vi "indicator.vi"(0 "Dial":i8(knob) scale=0.0..9.0, 1 "Boolean 9":bool) -> ()   [LabVIEW 2022 SP3]
panel:
  in  "stop":bool
  out "Boolean 8":bool
  out "Boolean 7":bool
  out "Boolean 6":bool
  out "Boolean 5":bool
  out "Boolean 4":bool
  out "Boolean 3":bool
  out "Boolean 2":bool
  out "Boolean":bool
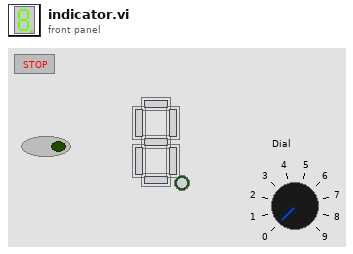
[diagram p1: front panel]
types:
  T1 = cluster{bool, bool, bool, bool, bool, bool, bool}
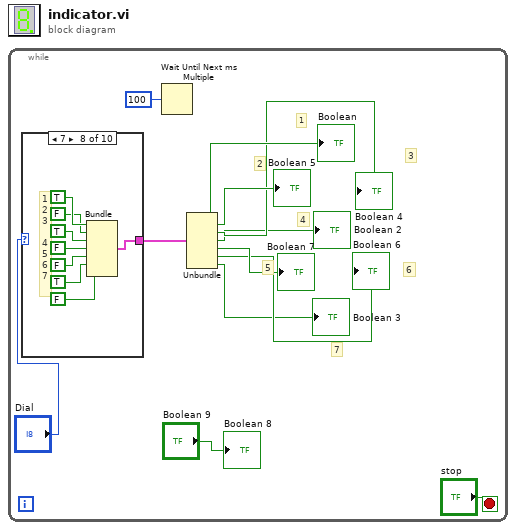
[diagram p0: block diagram]
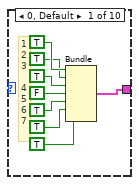
[diagram p2: hidden frame]
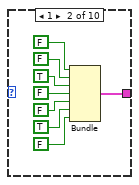
[diagram p3: hidden frame]
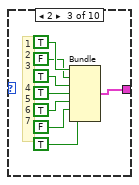
[diagram p4: hidden frame]
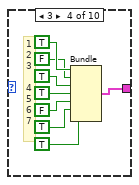
[diagram p5: hidden frame]
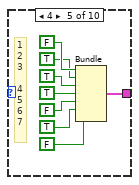
[diagram p6: hidden frame]
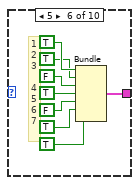
[diagram p7: hidden frame]
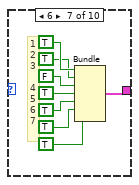
[diagram p8: hidden frame]
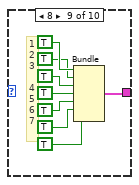
[diagram p9: hidden frame]
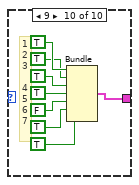
[diagram p10: hidden frame]
diagram:
  n1 = while {
    stop <- "stop" stop-if-true
    # "7"
    # "6"
    # "5"
    # "4"
    # "3"
    # "2"
    # "1"
    n2 = case shown="7" "Dial" {
      tunnel: [w13 w21 w29 w37 w45 w53 w61 w69 w77 w85] -> w12
      frame 0, Default {
        # "1\n2\n3\n\n4\n5\n6\n7"
        n3 = Bundle(TRUE, TRUE, TRUE, FALSE, TRUE, TRUE, TRUE) -> (w13:T1)  [unwired: 1 in]
      }
      frame 1 {
        n4 = Bundle(FALSE, FALSE, TRUE, FALSE, FALSE, TRUE, FALSE) -> (w21:T1)  [unwired: 1 in]
      }
      frame 2 {
        # "1\n2\n3\n\n4\n5\n6\n7"
        n5 = Bundle(TRUE, FALSE, TRUE, TRUE, TRUE, FALSE, TRUE) -> (w29:T1)  [unwired: 1 in]
      }
      frame 3 {
        # "1\n2\n3\n\n4\n5\n6\n7"
        n6 = Bundle(TRUE, FALSE, TRUE, TRUE, FALSE, TRUE, TRUE) -> (w37:T1)  [unwired: 1 in]
      }
      frame 4 {
        # "1\n2\n3\n\n4\n5\n6\n7"
        n7 = Bundle(FALSE, TRUE, TRUE, TRUE, FALSE, TRUE, FALSE) -> (w45:T1)  [unwired: 1 in]
      }
      frame 5 {
        # "1\n2\n3\n\n4\n5\n6\n7"
        n8 = Bundle(TRUE, TRUE, FALSE, TRUE, FALSE, TRUE, TRUE) -> (w53:T1)  [unwired: 1 in]
      }
      frame 6 {
        # "1\n2\n3\n\n4\n5\n6\n7"
        n9 = Bundle(TRUE, TRUE, FALSE, TRUE, TRUE, TRUE, TRUE) -> (w61:T1)  [unwired: 1 in]
      }
      frame 7 {
        # "1\n2\n3\n\n4\n5\n6\n7"
        n10 = Bundle(TRUE, FALSE, TRUE, FALSE, FALSE, TRUE, FALSE) -> (w69:T1)  [unwired: 1 in]
      }
      frame 8 {
        # "1\n2\n3\n\n4\n5\n6\n7"
        n11 = Bundle(TRUE, TRUE, TRUE, TRUE, TRUE, TRUE, TRUE) -> (w77:T1)  [unwired: 1 in]
      }
      frame 9 {
        # "1\n2\n3\n\n4\n5\n6\n7"
        n12 = Bundle(TRUE, TRUE, TRUE, TRUE, FALSE, TRUE, TRUE) -> (w85:T1)  [unwired: 1 in]
      }
    }
    n13 = Wait Until Next ms Multiple(millisecond multiple=u32 100) -> ()  [unwired: 1 out]
    n14 = Unbundle(w12) -> (→"Boolean":bool, →"Boolean 5":bool, →"Boolean 4":bool, →"Boolean 2":bool, →"Boolean 7":bool, →"Boolean 6":bool, →"Boolean 3":bool)
    "Boolean 8" <- "Boolean 9"
  }
